vi "专用-遍历扫描网络探头.vi"(8 "发现的探头[]-引用":refnum<vi>, 9 "扫描结果-引用":refnum<vi>, 10 "扫描进度-引用":refnum<vi>, 11 "忙碌VI":refnum<vi>) -> ()   [LabVIEW 2017]
panel:
  out "模块IP与MAC":cluster{"IP":string, "MAC":string}[](array[cluster])
  out "保存过的网口探头":string[](array[string])
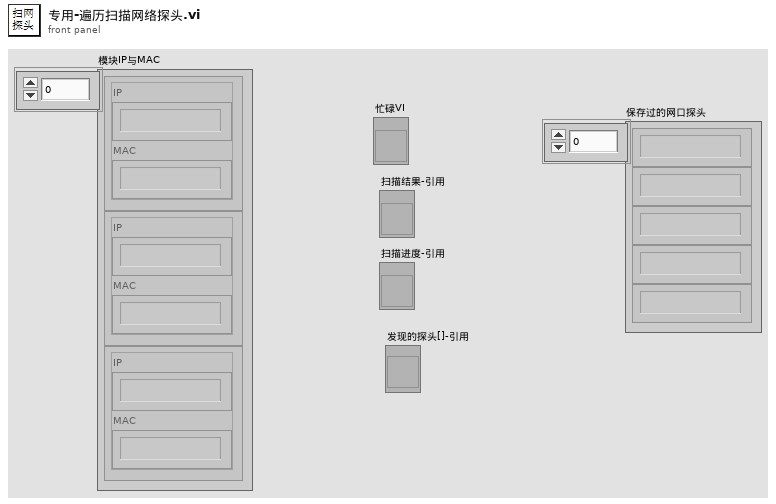
[diagram p1: front panel]
types:
  T1 = typedef "探测器信息.ctl" = cluster{"网络地址":string, "名称":string, "备注":string, "累积剂量":dbl, "累积限值":dbl, "硬件剂量率限值":T2, "剂量率限值1":dbl, "剂量率限值2":dbl, "报警方式":T3}
  T2 = typedef "探头剂量率限值选择.ctl" = enum16{"一级限值", "二级限值"}
  T3 = typedef "报警方式选择.ctl" = enum16{"常报警", "自动静音", "手动静音"}
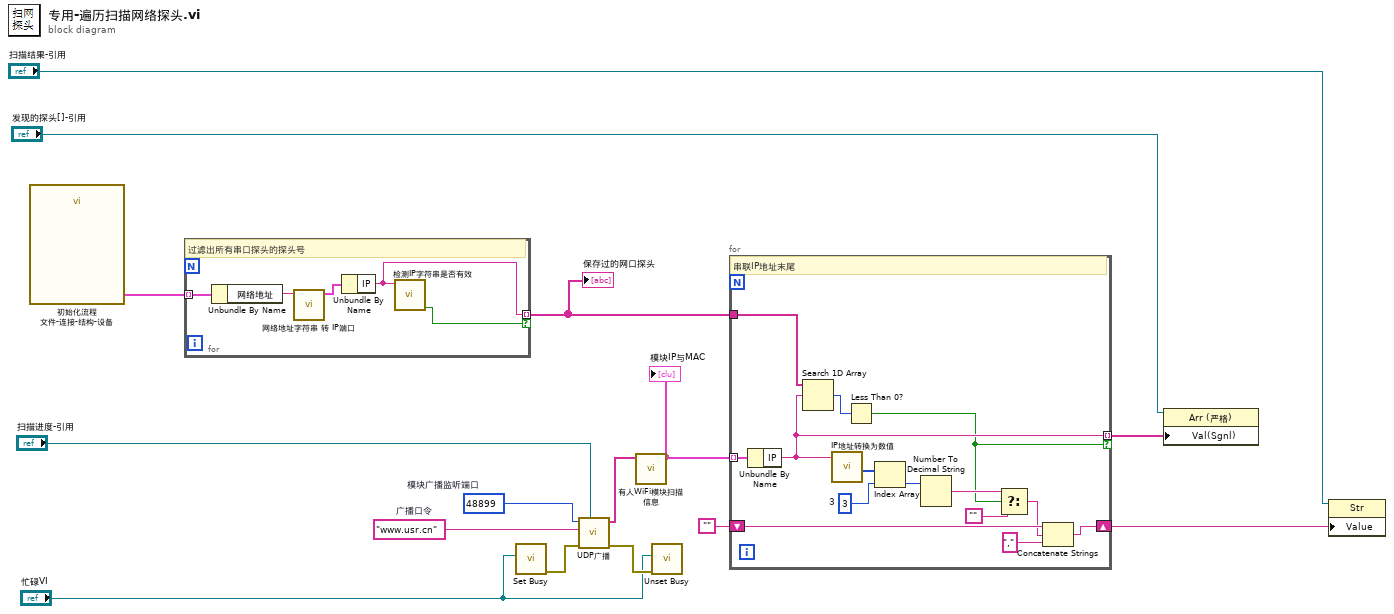
[diagram p0: block diagram]
diagram:
  w9 = "www.usr.cn"  # 广播口令
  w8 = u16 48899  # 模块广播监听端口
  n1 = call "初始化流程 文件-连接-结构-设备.vi"() -> ("探测器信息[]"=w15:T1[])  [unwired: 10 in, 1 out]
  n2 = for {
    tunnel: w15 -> [w20] mode=indexing
    tunnel: [w16] -> w3 mode=indexing if=w17
    # "过滤出所有串口探头的探头号"
    n3 = Unbundle By Name(w20) -> ("网络地址"=w18:string)
    n4 = call "网络地址字符串 转 IP端口.vi"("IP端口字符串"=w18) -> ("IP端口"=w19:cluster{"IP":string, "Port":u16})  [unwired: 10 in]
    n5 = Unbundle By Name(w19) -> ("IP"=w16:string)
    n6 = call "检测IP字符串是否有效.vi"("IP地址"=w16) -> ("有效IP？"=w17:bool)  [unwired: 10 in]
  }
  "保存过的网口探头" <- w3
  n7 = call <vilib>:"Set Busy.vi"("VI reference (current VI)"="忙碌VI") -> ("error out"=w10:errorcluster)  [unwired: 9 in, 1 out]
  n8 = call "UDP广播.vi"("文本控件"="扫描进度-引用", "错误输入（无错误）"=w10, "数据输入"=w9, "端口或服务名称"=w8) -> ("error out"=w11:errorcluster, "接收"=w14:string[])  [unwired: 6 in]
  n9 = call "有人WiFi模块扫描信息.vi"("扫描广播回复"=w14) -> ("模块IP与MAC"=w12:cluster{"IP":string, "MAC":string}[])  [unwired: 9 in, 1 out]
  "模块IP与MAC" <- w12
  n10 = call <vilib>:"Unset Busy.vi"("error in (no error)"=w11, "VI reference (current VI)"="忙碌VI") -> ()  [unwired: 9 in, 1 out]
  n11 = for {
    tunnel: w12 -> [w33] mode=indexing
    shift-right: [w31] -> w5
    shift-left: "" -> [w34]
    tunnel: w3 -> [w27]
    tunnel: [w22] -> w1 mode=indexing if=w21
    w29 = 3  # 3
    # "串联IP地址末尾"
    n12 = Unbundle By Name(w33) -> ("IP"=w22:string)
    n13 = Search 1D Array(1D array=w27, element=w22) -> (index of element=w26:i32)  [unwired: 1 in]
    n14 = call "IP地址转换为数值.vi"("IP地址"=w22) -> ("数组"=w30:u8[])  [unwired: 8 in, 2 out]
    n15 = Less Than 0?(x=w26) -> (x < 0?=w21:bool)
    n16 = Index Array(array=w30, index=w29) -> (element=w28:u8)
    n17 = Number To Decimal String(number=w28) -> (decimal integer string=w24:string)  [unwired: 1 in]
    n18 = Select(t=w24, s=w21, f="") -> (s? t:f=w23:string)
    n19 = Concatenate Strings(w34, w23, "," ("字符串")) -> (w31:string)
  }
  n20 = property on="属性节点" class="Arr (严格)"(reference="发现的探头[]-引用", "Val(Sgnl)"=w1) -> ()  [unwired: 1 in, 2 out]
  n21 = property class="Str"(reference="扫描结果-引用", "Value"=w5) -> ()  [unwired: 1 in, 2 out]
